vi "Puzzle 5-2.vi"() -> ()   [LabVIEW 2022 SP3]
panel:
  in  "delimited string":string
  out "Waveform Graph":i64[](graph)
  out "Waveform Graph 2":i64[](graph)
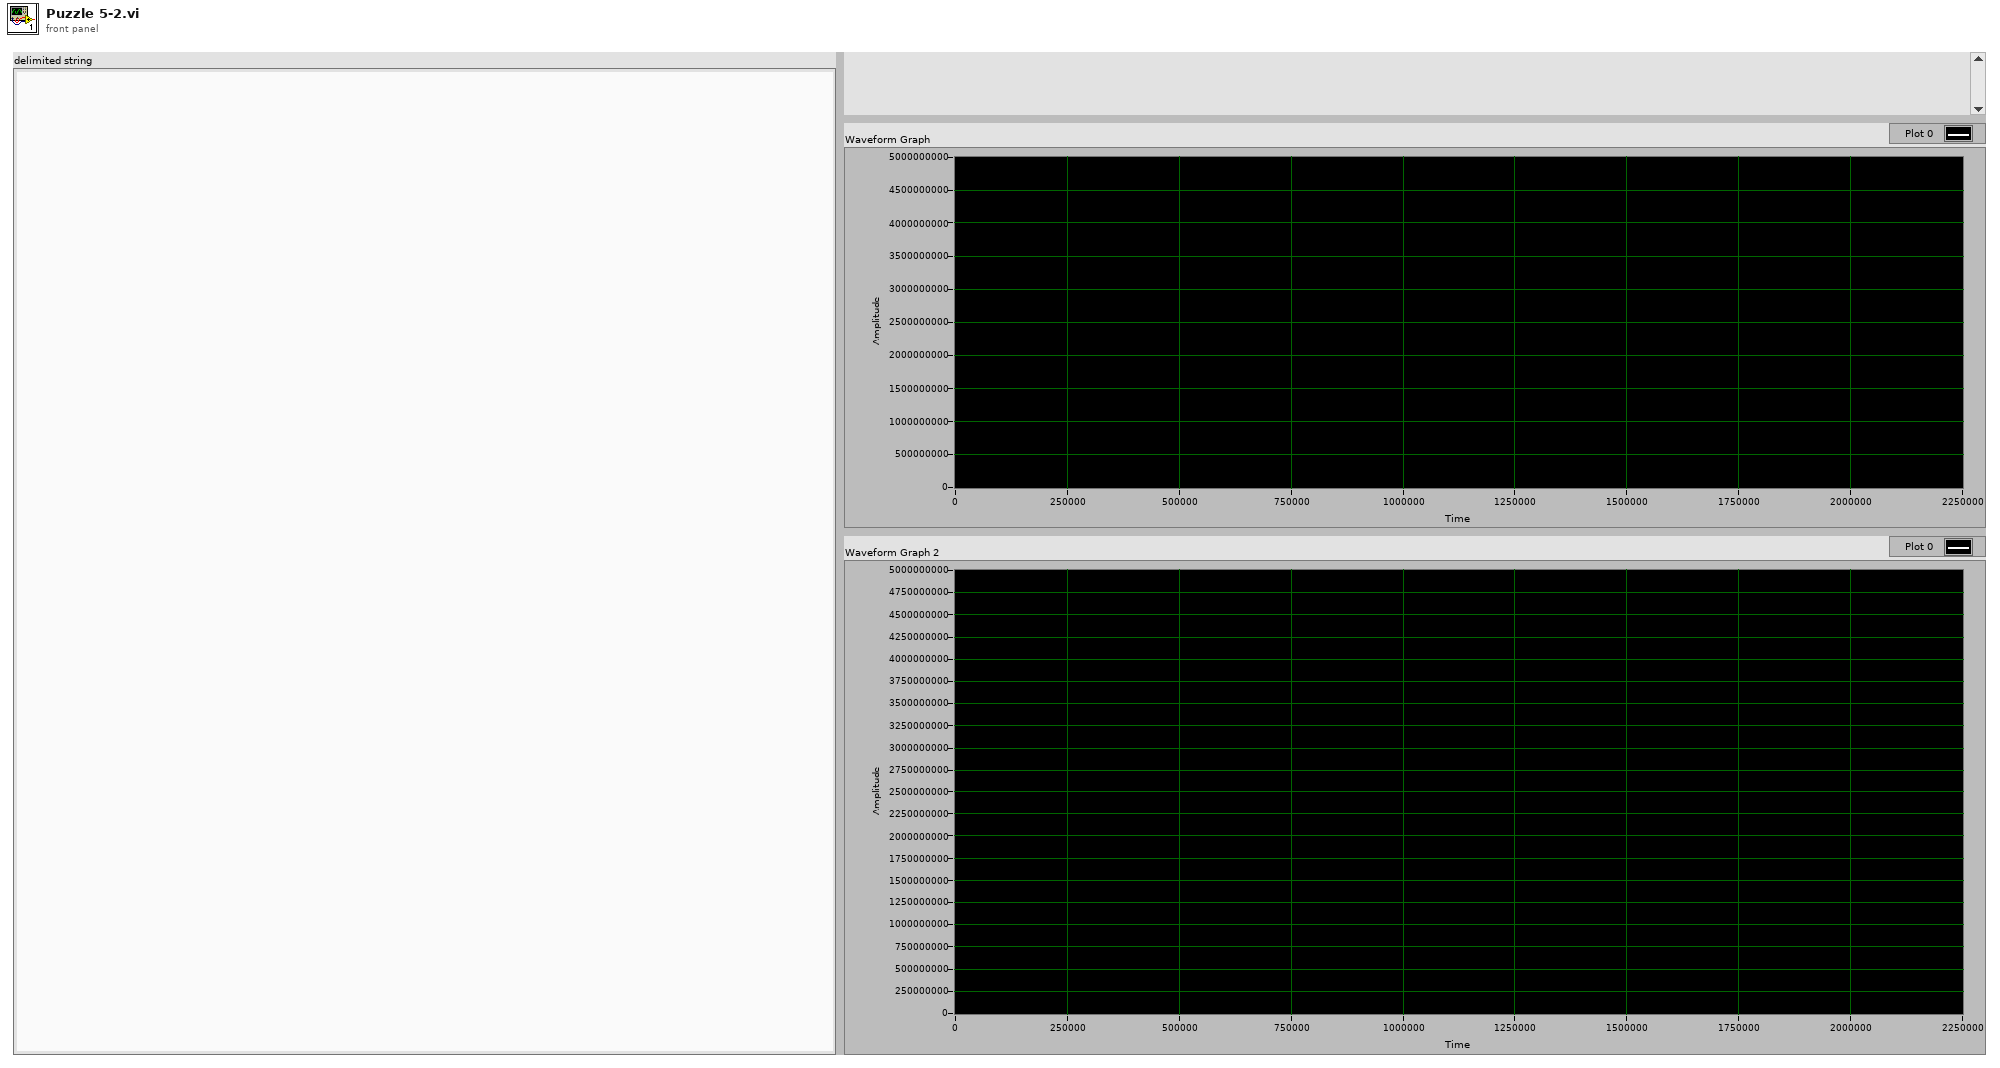
[diagram p1: front panel]
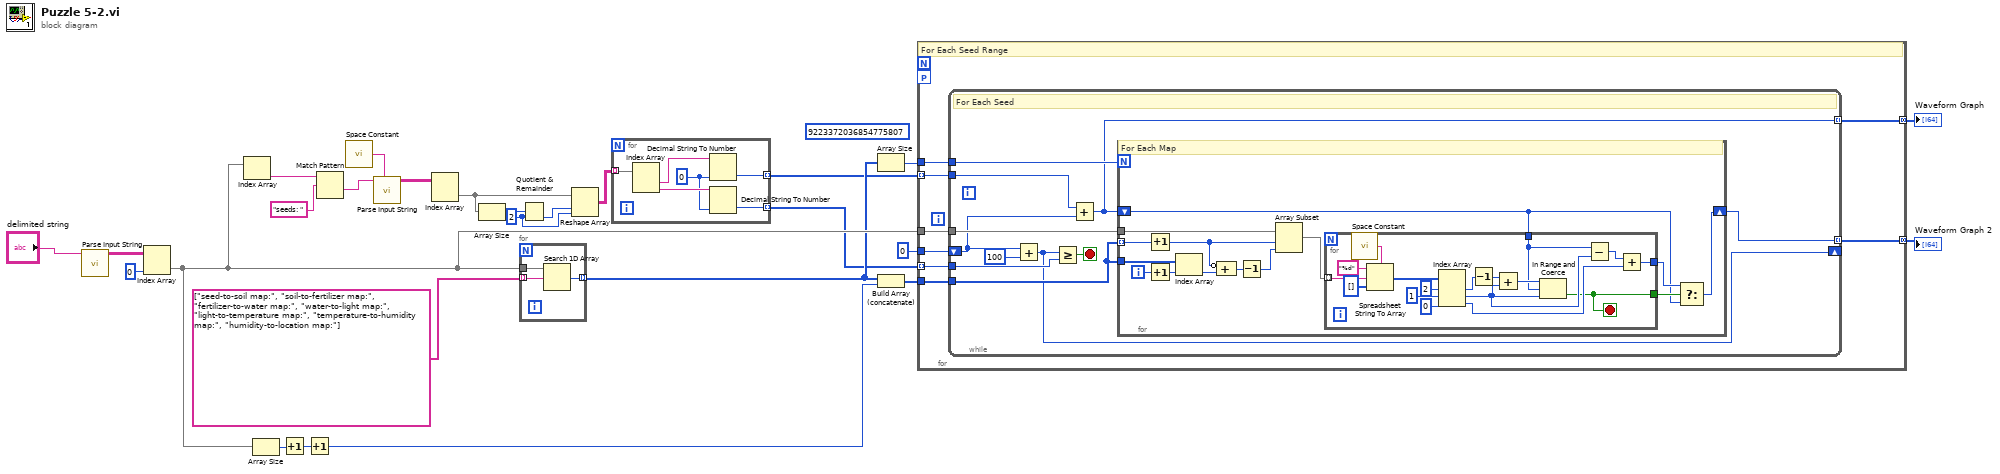
[diagram p0: block diagram]
diagram:
  (unwired) i64 9223372036854775807
  w7 = 2 ("y")
  n1 = call "Parse Input String.vi"("delimited string"="delimited string") -> ("parsed string"=w26:string[][])  [unwired: 10 in]
  n2 = Index Array(array=w26, index (col)=0 ("disabled index (col)")) -> (element=w17:string[])  [unwired: 1 in]
  n3 = Index Array(array=w17) -> (element=w22:string)  [unwired: 1 in]
  n4 = Array Size(array=w17) -> (size(s)=w16:i32)
  n5 = Increment(x=w16) -> (x+1=w15:i32)
  n6 = Increment(x=w15) -> (x+1=w14:i32)
  n7 = Match Pattern(string=w22, regular expression="seeds: " ("format string")) -> (after substring=w20:string)  [unwired: 1 in, 3 out]
  n8 = call <vilib>:"Space Constant.vi"() -> ("String"=w23:string)
  n9 = call "Parse Input String.vi"("delimiter (Tab)"=w23, "delimited string"=w20) -> ("parsed string"=w18:string[][])  [unwired: 9 in]
  n10 = Index Array(array=w18) -> (element=w10:string[])  [unwired: 2 in]
  n11 = Array Size(array=w10) -> (size(s)=w9:i32)
  n12 = for {
    tunnel: w17 -> [w29]
    tunnel: string[] ["seed-to-soil map:", "soil-to-fertilizer map:", "fertilizer-to-water map:", "water-to-light map:", "light-to-temperature map:", "temperature-to-humidity map:", "humidity-to-location map:"] ("subarray") -> [w28] mode=indexing
    tunnel: [w27] -> w12 mode=indexing
    n13 = Search 1D Array(1D array=w29, element=w28) -> (index of element=w27:i32)  [unwired: 1 in]
  }
  n14 = Quotient & Remainder(x=w9, y=w7) -> (floor(x/y)=w8:i32)  [unwired: 1 out]
  n15 = Reshape Array(w10, w8, w7) -> (w6:string[][])
  n16 = for {
    tunnel: w6 -> [w35] mode=indexing
    tunnel: [w31] -> w4 mode=indexing
    tunnel: [w30] -> w5 mode=indexing
    w32 = i64 0 ("default (0 I32)")
    n17 = Index Array(array=w35) -> (element #1=w34:string, element #2=w33:string)  [unwired: 2 in]
    n18 = Decimal String To Number(string=w34, default (0L)=w32) -> (number=w30:i64)  [unwired: 1 in, 1 out]
    n19 = Decimal String To Number(string=w33, default (0L)=w32) -> (number=w31:i64)  [unwired: 1 in, 1 out]
  }
  n20 = Array Size(array=w12) -> (size(s)=w11:i32)
  n21 = Build Array (concatenate)(w12, w14) -> (w13:i32[])
  n22 = for {
    tunnel: w17 -> [w43]
    tunnel: w13 -> [w42]
    tunnel: w11 -> [w41]
    tunnel: w5 -> [w40] mode=indexing
    tunnel: w4 -> [w39] mode=indexing
    tunnel: i64 0 -> [w38]
    tunnel: [w37] -> w2 mode=concatenating
    tunnel: [w36] -> w1 mode=concatenating
    workers-P: _ -> [_]
    # "For Each Seed Range"
    n23 = while {
      tunnel: w43 -> [w54]
      tunnel: w42 -> [w49]
      tunnel: w41 -> [w53]
      tunnel: w40 -> [w52]
      tunnel: w39 -> [w51]
      shift-right: [w44] -> _
      shift-left: w38 -> [w48]
      tunnel: [w46] -> w37 mode=indexing
      tunnel: [w45] -> w36 mode=indexing
      stop <- w50 stop-if-true
      # "For Each Seed"
      n24 = Add(x=w48, y=i64 100) -> (x+y=w44:i64)
      n25 = Greater Or Equal?(x=w44, y=w51) -> (x >= y?=w50:bool)
      n26 = Add(x=w52, y=w48) -> (x+y=w46:i64)
      n27 = for {
        N: w53 -> [_]
        tunnel: w54 -> [w68]
        tunnel: w49 -> [w64] mode=indexing
        shift-right: [w55] -> w45
        shift-left: w46 -> [w56]
        tunnel: w49 -> [w65]
        i -> [w67]
        # "For Each Map"
        n28 = Increment(x=w64) -> (x+1=w62:i32)
        n29 = Increment(x=w67) -> (x+1=w66:i32)
        n30 = Index Array(array=w65, index=w66) -> (element=w61:i32)
        n31 = Compound Arithmetic op=ADD(invert w62, w61) -> (w60:i32)
        n32 = Decrement(x=w60) -> (x-1=w63:i32)
        n33 = Array Subset(array=w68, index=w62, length=w63) -> (w59:string[])
        n34 = for {
          tunnel: w59 -> [w85] mode=indexing
          tunnel: w56 -> [w74]
          tunnel: [w70] -> w58
          tunnel: [w69] -> w57
          stop <- w70 stop-if-true
          n35 = call <vilib>:"Space Constant.vi"() -> ("String"=w82:string)
          n36 = Spreadsheet String To Array(delimiter (Tab)=w82, format string="%d", spreadsheet string=w85, array type (2D Dbl)=i64[] []) -> (array=w81:i64[])
          n37 = Index Array(array=w81, index #1=2 ("index"), index #2=1 ("index"), index #3=0 ("index")) -> (element #1=w78:i64, element #2=w73:i64, element #3=w71:i64)
          n38 = Decrement(x=w78) -> (x-1=w77:i64)
          n39 = Add(x=w77, y=w73) -> (x+y=w76:i64)
          n40 = In Range and Coerce(upper limit=w76, x=w74, lower limit=w73) -> (In Range?=w70:bool)  [unwired: 1 out]
          n41 = Subtract(x=w74, y=w73) -> (x-y=w72:i64)
          n42 = Add(x=w72, y=w71) -> (x+y=w69:i64)
        }
        n43 = Select(t=w57, s=w58, f=w56) -> (s? t:f=w55:i64)
      }
    }
  }
  "Waveform Graph" <- w2
  "Waveform Graph 2" <- w1
